vi "Result.vi"(7 "MainProcess":T1=enum."SystemInit", 9 "Result":bool, 11 "Result":refnum<vi>) -> (3 "Result":refnum<vi>)   [LabVIEW 2013]
uses:
  Control/SystemProcess.ctl
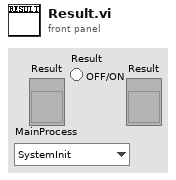
[diagram p1: front panel]
types:
  T1 = typedef "SystemProcess.ctl" = enum16{"Idle", "SystemInit", "SpecialEvent", "Barcode(SN)", "TestInitialize", "Test", "Stop", "SaveTestData", "Exit"}
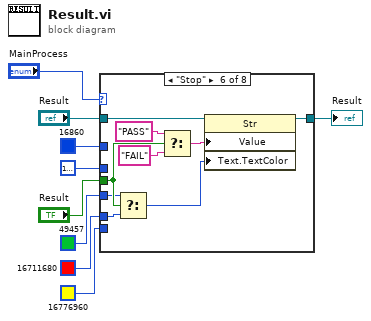
[diagram p0: block diagram]
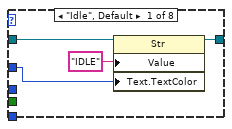
[diagram p2: hidden frame]
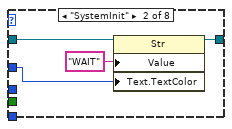
[diagram p3: hidden frame]
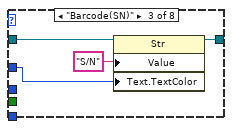
[diagram p4: hidden frame]
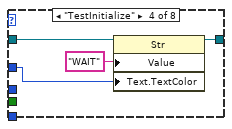
[diagram p5: hidden frame]
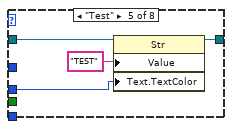
[diagram p6: hidden frame]
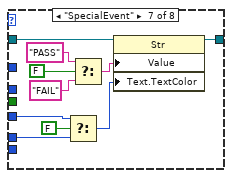
[diagram p7: hidden frame]
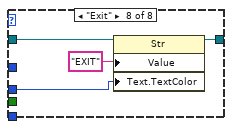
[diagram p8: hidden frame]
diagram:
  n1 = case shown="\"Stop\"" "MainProcess" {
    tunnel: [w11 w15 w19 w23 w27 w37 w44 w49] -> w9
    tunnel: "Result" -> [w12 w16 w20 w24 w28 w38 w43 w50]
    tunnel: u32 16860 -> [w10 w14 w18 w22 _ _ _ _]
    tunnel: u32 16777228 -> [_ _ _ _ w26 _ _ w51]
    tunnel: u32 16776960 -> [_ _ _ _ _ _ _ _]
    tunnel: u32 49457 -> [_ _ _ _ _ w32 w42 _]
    tunnel: u32 16711680 -> [_ _ _ _ _ w31 w41 _]
    tunnel: "Result" -> [_ _ _ _ _ w33 _ _]
    frame "Idle", Default {
      n2 = property class="Str"(reference=w12, "Value"="IDLE", "Text.TextColor"=w10) -> (reference out=w11:refnum<vi>)  [unwired: 1 in, 1 out]
    }
    frame "SystemInit" {
      n3 = property class="Str"(reference=w16, "Value"="WAIT", "Text.TextColor"=w14) -> (reference out=w15:refnum<vi>)  [unwired: 1 in, 1 out]
    }
    frame "Barcode(SN)" {
      n4 = property class="Str"(reference=w20, "Value"="S/N", "Text.TextColor"=w18) -> (reference out=w19:refnum<vi>)  [unwired: 1 in, 1 out]
    }
    frame "TestInitialize" {
      n5 = property class="Str"(reference=w24, "Value"="WAIT", "Text.TextColor"=w22) -> (reference out=w23:refnum<vi>)  [unwired: 1 in, 1 out]
    }
    frame "Test" {
      n6 = property class="Str"(reference=w28, "Value"="TEST", "Text.TextColor"=w26) -> (reference out=w27:refnum<vi>)  [unwired: 1 in, 1 out]
    }
    frame "Stop" {
      n7 = Select(t=w32, s=w33, f=w31) -> (s? t:f=w30:u32)
      n8 = Select(t="PASS", s=w33, f="FAIL") -> (s? t:f=w36:string)
      n9 = property class="Str"(reference=w38, "Value"=w36, "Text.TextColor"=w30) -> (reference out=w37:refnum<vi>)  [unwired: 1 in, 1 out]
    }
    frame "SpecialEvent" {
      n10 = Select(t=w42, s=FALSE, f=w41) -> (s? t:f=w48:u32)
      n11 = Select(t="PASS", s=FALSE, f="FAIL" ("Value")) -> (s? t:f=w47:string)
      n12 = property class="Str"(reference=w43, "Value"=w47, "Text.TextColor"=w48) -> (reference out=w44:refnum<vi>)  [unwired: 1 in, 1 out]
    }
    frame "Exit" {
      n13 = property class="Str"(reference=w50, "Value"="EXIT", "Text.TextColor"=w51) -> (reference out=w49:refnum<vi>)  [unwired: 1 in, 1 out]
    }
  }
  "Result" <- w9
